vi "DisplayValuesFromPLC.vi"(0 "Input Registers":u16[](array[numeric])) -> (3 "output array":string[][](array[string]), 4 "Error":bool, 5 "String":string, 6 "Boolean 1":bool, 7 "Boolean 14":bool, 8 "Boolean 2":bool, 9 "Boolean 13":bool, 10 "Boolean 3":bool, 11 "Boolean 12":bool, 12 "Boolean 4":bool, 13 "Boolean 11":bool, 14 "Boolean 5":bool, 15 "Boolean 6":bool, 16 "Boolean 7":bool, 17 "Boolean 8":bool, 18 "Boolean 9":bool, 19 "Boolean 10":bool)   [LabVIEW 2020, in "Modbus.lvlib"]
uses:
  Modbus/Modbus.lvlib
panel:
  out "subarray":u16[](array[numeric])
  out "number of rows":i32
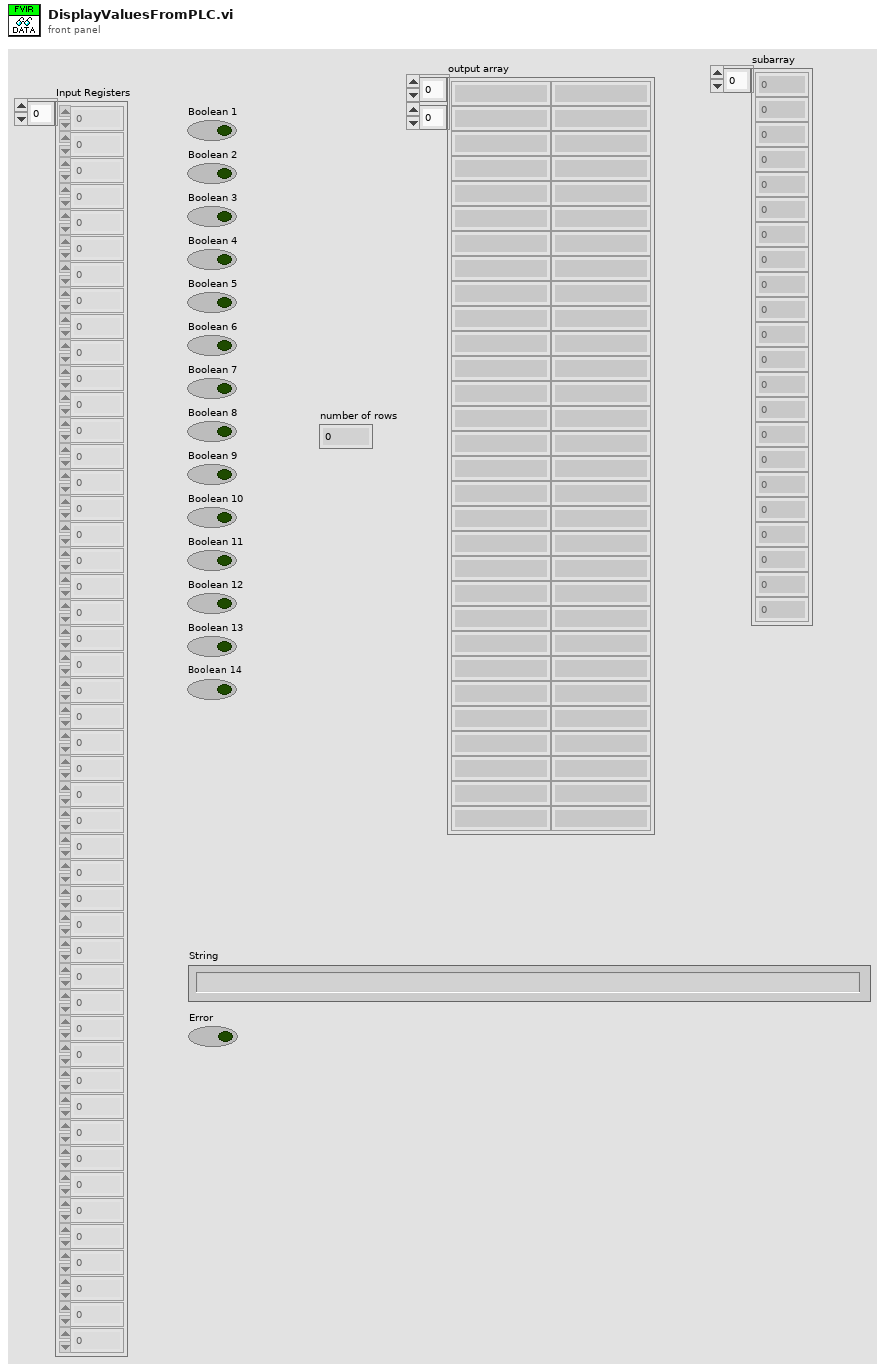
[diagram p1: front panel]
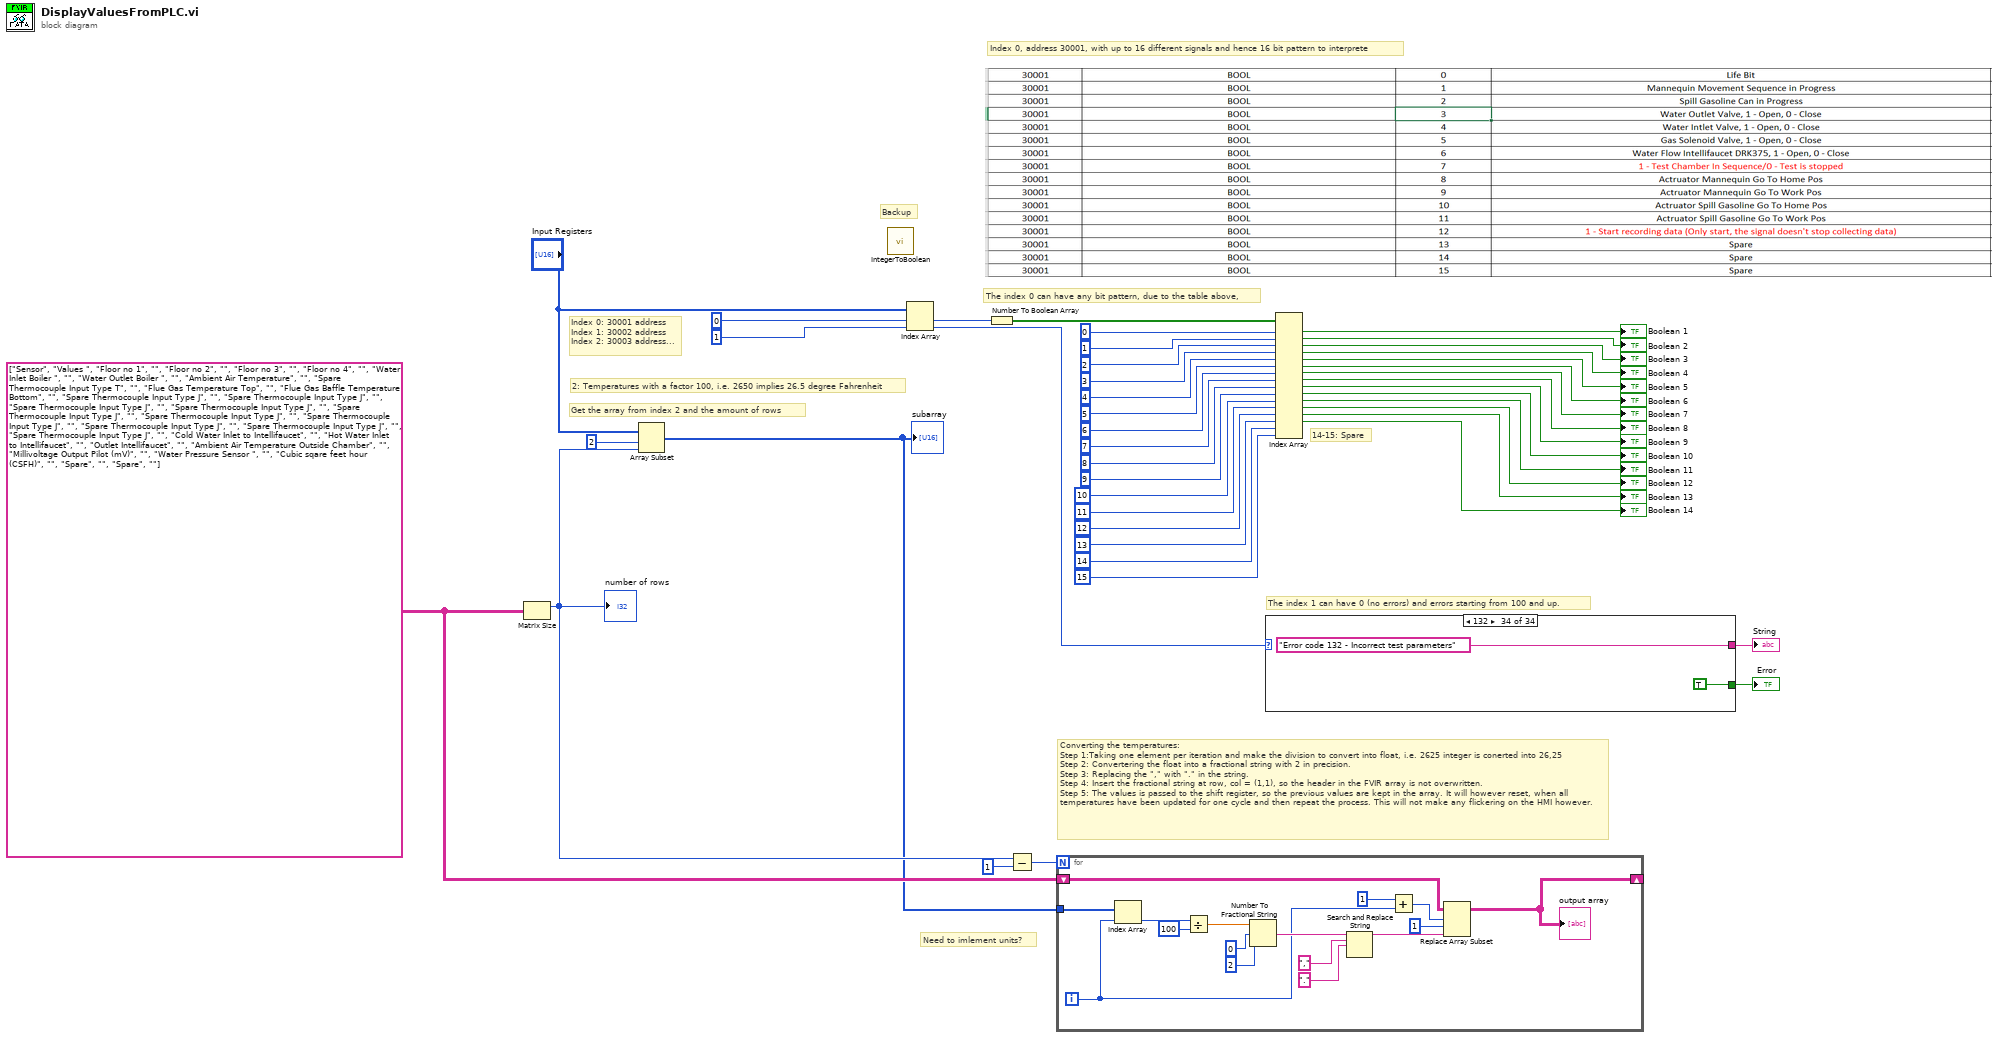
[diagram p0: block diagram]
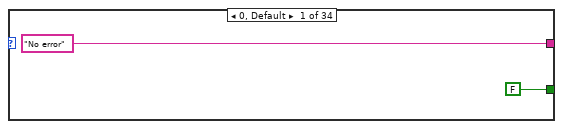
[diagram p2: hidden frame]
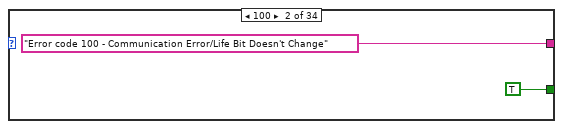
[diagram p3: hidden frame]
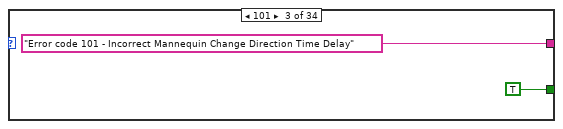
[diagram p4: hidden frame]
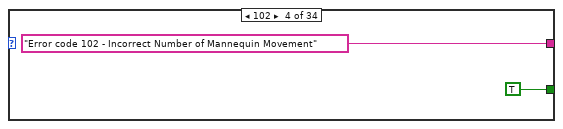
[diagram p5: hidden frame]
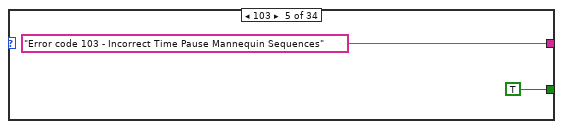
[diagram p6: hidden frame]
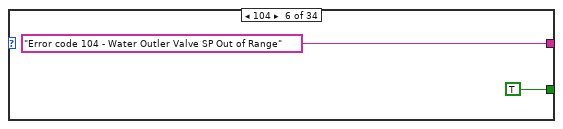
[diagram p7: hidden frame]
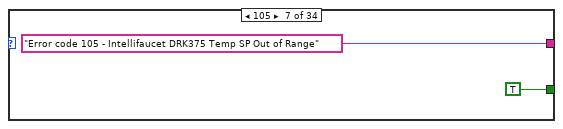
[diagram p8: hidden frame]
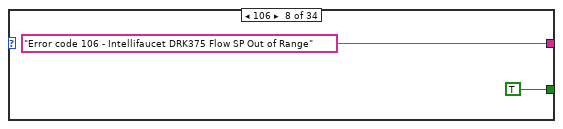
[diagram p9: hidden frame]
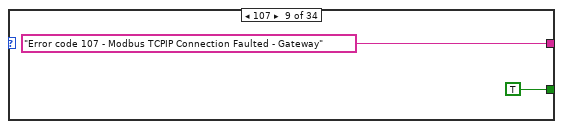
[diagram p10: hidden frame]
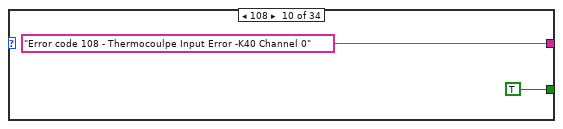
[diagram p11: hidden frame]
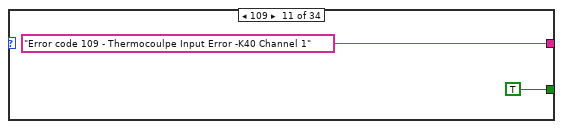
[diagram p12: hidden frame]
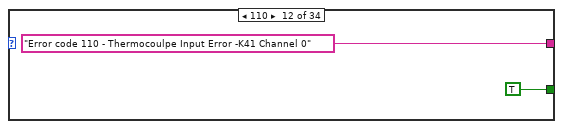
[diagram p13: hidden frame]
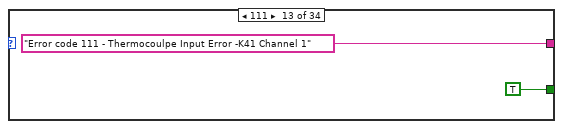
[diagram p14: hidden frame]
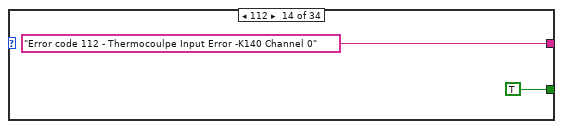
[diagram p15: hidden frame]
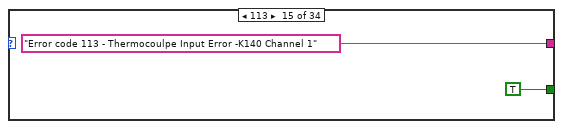
[diagram p16: hidden frame]
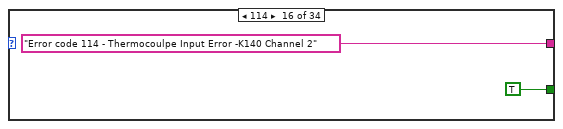
[diagram p17: hidden frame]
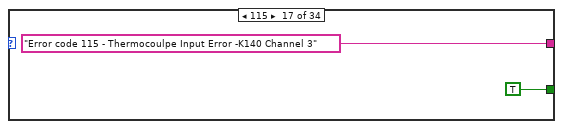
[diagram p18: hidden frame]
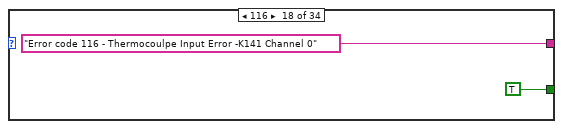
[diagram p19: hidden frame]
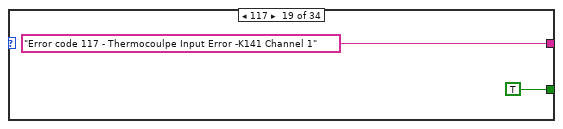
[diagram p20: hidden frame]
diagram:
  w23 = string[][] [["Sensor", "Values "], ["Floor no 1", ""], ["Floor no 2", ""], ["Floor no 3", ""], ["Floor no 4", ""], ["Water Inlet Boiler ", ""], ["Water Outlet Boiler ", ""], ["Ambient Air Temperature", ""], ["Spare Thermocouple Input Type T", ""], ["Flue Gas Temperature Top", ""], ["Flue Gas Baffle Temperature Bottom", ""], ["Spare Thermocouple Input Type J", ""], ["Spare Thermocouple Input Type J", ""], ["Spare Thermocouple Input Type J", ""], ["Spare Thermocouple Input Type J", ""], ["Spare Thermocouple Input Type J", ""], ["Spare Thermocouple Input Type J", ""], ["Spare Thermocouple Input Type J", ""], ["Spare Thermocouple Input Type J", ""], ["Spare Thermocouple Input Type J", ""], ["Spare Thermocouple Input Type J", ""], ["Cold Water Inlet to Intellifaucet", ""], ["Hot Water Inlet to Intellifaucet", ""], ["Outlet Intellifaucet", ""], ["Ambient Air Temperature Outside Chamber", ""], ["Millivoltage Output Pilot (mV)", ""], ["Water Pressure Sensor ", ""], ["Cubic sqare feet hour (CSFH)", ""], ["Spare", ""], ["Spare", ""]] ("Array 2")
  # "Index 0, address 30001, with up to 16 different signals and hence 16 bit pattern to interprete"
  # "Index 0: 30001 address\nIndex 1: 30002 address\nIndex 2: 30003 address..."
  # "The index 0 can have any bit pattern, due to the table above,"
  # "Backup"
  # "Converting the temperatures: \nStep 1:Taking one element per iteration and make the division to convert into float, i.e. 2625 integer is conerted into 26,25\nStep 2: Convertering the float into a fractional string with 2 in precision. \nStep 3: Replacing the \",\" with \".\" in the string.\nStep 4: Insert the fractional string at row, col = (1,1), so the header in the FVIR array is not overwritten. \nStep 5: The values is passed to the shift register, so the previous values are kept in the array. It will however reset, when all temperatures have been updated for one cycle and then repeat the process. This will not make any flickering on the HMI however."
  # "Get the array from index 2 and the amount of rows"
  # "Need to imlement units?"
  # "2: Temperatures with a factor 100, i.e. 2650 implies 26.5 degree Fahrenheit"
  # "The index 1 can have 0 (no errors) and errors starting from 100 and up."
  # "14-15: Spare"
  n1 = Matrix Size(0:w23) -> (1:w22:i32)  [unwired: 1 out]
  "number of rows" <- w22
  n2 = Array Subset(array="Input Registers", index=2, length=w22) -> (w2:u16[])
  "subarray" <- w2
  n3 = call "IntegerToBoolean.vi"() -> ()  [unwired: 11 in, 1 out]
  n4 = Index Array(array="Input Registers", index #1=0 ("index"), index #2=1 ("index")) -> (element #1=w5:u16, element #2=w4:u16)
  n5 = Number To Boolean Array(number=w5) -> (Boolean array=w19:bool[])
  n6 = Subtract(x=w22, y=1) -> (x-y=w26:i32)
  n7 = for {
    N: w26 -> [_]
    tunnel: w2 -> [w55]
    shift-right: [w50] -> _
    shift-left: w23 -> [w49]
    i -> [w47]
    n8 = Index Array(array=w55, index=w47) -> (element=w46:u16)
    n9 = Divide(x=w46, y=u16 100) -> (x/y=w45:dbl)
    n10 = Number To Fractional String(number=w45, width (-)=i16 0, precision (6)=i16 2) -> (F-format string=w57:string)  [unwired: 1 in]
    n11 = Search and Replace String(input string=w57, search string=",", replace string="." ("replace string (\"\")")) -> (result string=w53:string)  [unwired: 5 in, 3 out]
    n12 = Add(x=1, y=w47) -> (x+y=w51:i32)
    n13 = Replace Array Subset(array=w49, new element=w53, index (row)=w51, index (col)=1) -> (w50:string[][])
    "output array" <- w50
  }
  n14 = case shown="132" w4 {
    tunnel: ["No error" "Error code 100 - Communication Error/Life Bit Doesn't Change" "Error code 101 - Incorrect Mannequin Change Direction Time Delay" "Error code 102 - Incorrect Number of Mannequin Movement" "Error code 103 - Incorrect Time Pause Mannequin Sequences" "Error code 104 - Water Outler Valve SP Out of Range" "Error code 105 - Intellifaucet DRK375 Temp SP Out of Range" "Error code 106 - Intellifaucet DRK375 Flow SP Out of Range" "Error code 107 - Modbus TCPIP Connection Faulted - Gateway" "Error code 108 - Thermocoulpe Input Error -K40 Channel 0" "Error code 109 - Thermocoulpe Input Error -K40 Channel 1" "Error code 110 - Thermocoulpe Input Error -K41 Channel 0" "Error code 111 - Thermocoulpe Input Error -K41 Channel 1" "Error code 112 - Thermocoulpe Input Error -K140 Channel 0" "Error code 113 - Thermocoulpe Input Error -K140 Channel 1" "Error code 114 - Thermocoulpe Input Error -K140 Channel 2" "Error code 115 - Thermocoulpe Input Error -K140 Channel 3" "Error code 116 - Thermocoulpe Input Error -K141 Channel 0" "Error code 117 - Thermocoulpe Input Error -K141 Channel 1" "Error code 118 - Thermocoulpe Input Error -K141 Channel 2" "Error code 119 - Thermocoulpe Input Error -K141 Channel 3" "Error code 120 - Thermocoulpe Input Error -K142 Channel 0" "Error code 121 - Thermocoulpe Input Error -K142 Channel 1" "Error code 122 - Thermocoulpe Input Error -K142 Channel 2" "Error code 123 - Thermocoulpe Input Error -K142 Channel 3" "Error code 124 - Thermocoulpe Input Error -K143 Channel 0" "Error code 125 - Thermocoulpe Input Error -K143 Channel 1" "Error code 126 - Thermocoulpe Input Error -K143 Channel 2" "Error code 127 - Thermocoulpe Input Error -K143 Channel 3" "Error code 128 - Thermocoulpe Input Error -K144 Channel 0" "Error code 129 - Thermocoulpe Input Error -K144 Channel 1" "Error code 130 - Thermocoulpe Input Error -K144 Channel 2" "Error code 131 - Thermocoulpe Input Error -K144 Channel 3" "Error code 132 - Incorrect test parameters"] -> w28
    tunnel: [FALSE TRUE TRUE TRUE TRUE TRUE TRUE TRUE TRUE TRUE TRUE TRUE TRUE TRUE TRUE TRUE TRUE TRUE TRUE TRUE TRUE TRUE TRUE TRUE TRUE TRUE TRUE TRUE TRUE TRUE TRUE TRUE TRUE TRUE] -> w27
    frame 0, Default {
    }
    frame 100 {
    }
    frame 101 {
    }
    frame 102 {
    }
    frame 103 {
    }
    frame 104 {
    }
    frame 105 {
    }
    frame 106 {
    }
    frame 107 {
    }
    frame 108 {
    }
    frame 109 {
    }
    frame 110 {
    }
    frame 111 {
    }
    frame 112 {
    }
    frame 113 {
    }
    frame 114 {
    }
    frame 115 {
    }
    frame 116 {
    }
    frame 117 {
    }
    frame 118 {
    }
    frame 119 {
    }
    frame 120 {
    }
    frame 121 {
    }
    frame 122 {
    }
    frame 123 {
    }
    frame 124 {
    }
    frame 125 {
    }
    frame 126 {
    }
    frame 127 {
    }
    frame 128 {
    }
    frame 129 {
    }
    frame 130 {
    }
    frame 131 {
    }
    frame 132 {
    }
  }
  "String" <- w28
  "Error" <- w27
  n15 = Index Array(array=w19, index #1=0 ("index"), index #2=1 ("index"), index #3=2 ("index"), index #4=3 ("index"), index #5=4 ("index"), index #6=5 ("index"), index #7=6 ("index"), index #8=7 ("index"), index #9=8 ("index"), index #10=9 ("index"), index #11=10 ("index"), index #12=11 ("index"), index #13=12 ("index"), index #14=13 ("index"), index #15=14 ("index"), index #16=15 ("index")) -> (element #1=→"Boolean 1":bool, element #2=→"Boolean 2":bool, element #3=→"Boolean 3":bool, element #4=→"Boolean 4":bool, element #5=→"Boolean 5":bool, element #6=→"Boolean 6":bool, element #7=→"Boolean 7":bool, element #8=→"Boolean 8":bool, element #9=→"Boolean 9":bool, element #10=→"Boolean 10":bool, element #11=→"Boolean 11":bool, element #12=→"Boolean 12":bool, element #13=→"Boolean 13":bool, element #14=→"Boolean 14":bool)  [unwired: 2 out]
